vi "Pixy Logic Core.vi"() -> ()   [LabVIEW 2016]
uses:
  Robot Global Data.vi
panel:
  out "Lcal Pixy Out (Y Axis)":dbl(graph)=25.833333333333332
  out "Value Rejection History":i16(graph)=1
  in  "Past array Width":dbl[](array[numeric])=[26.0, 26.0, 26.0, 25.0, 26.0, 26.0]
  in  "Y Axis Range":dbl=100.0
  out "Lcal Pixy Out (X Axis)":dbl(graph)=25.833333333333332
  # "Decoded Pixy Outputs are located in\n    \"Pixy1Or2ObjectSelection.vi\""
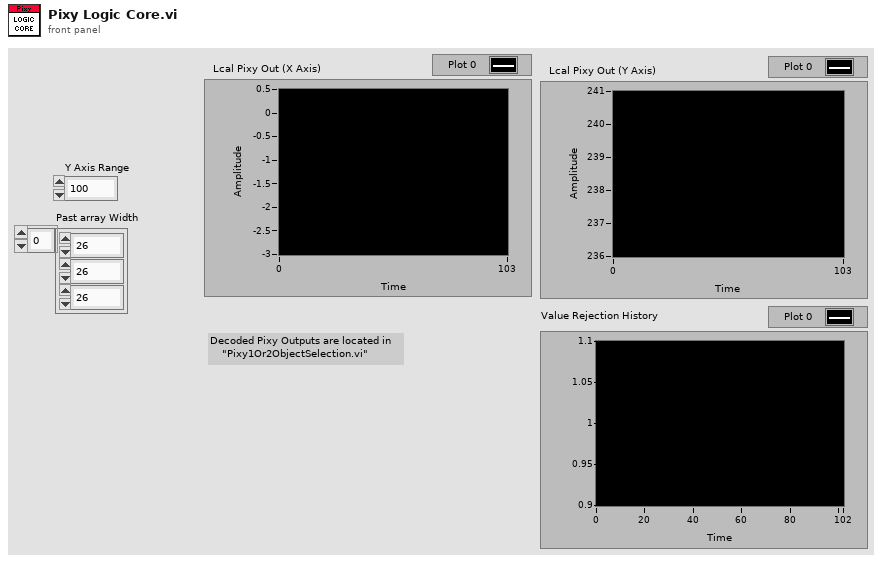
[diagram p1: front panel]
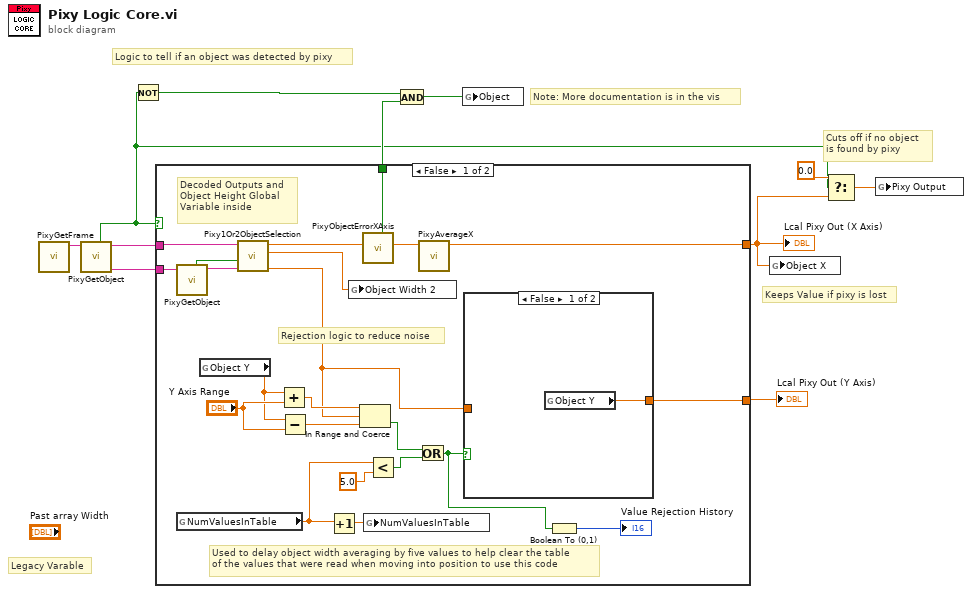
[diagram p0: block diagram]
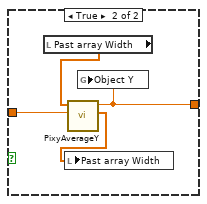
[diagram p2: hidden frame]
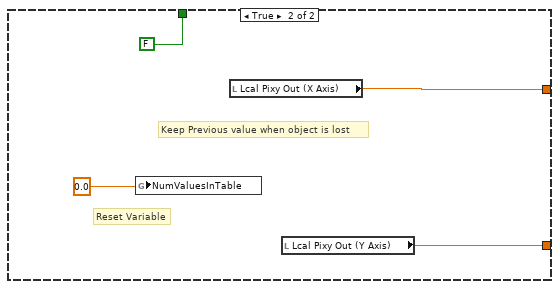
[diagram p3: hidden frame]
diagram:
  # "Note: More documentation is in the vis"
  # "Logic to tell if an object was detected by pixy"
  # "Legacy Varable"
  # "Keeps Value if pixy is lost"
  # "Cuts off if no object\nis found by pixy"
  n1 = call "PixyGetFrame.vi"() -> ("Frame"=w11:string)  [unwired: 11 in]
  n2 = call "PixyGetObject.vi"("Input Frame"=w11) -> ("Remainder of Frame"=w7:string, "Object"=w6:string, "Empty?"=w2:bool)  [unwired: 8 in]
  n3 = Not(x=w2) -> (.not. x?=w10:bool)
  n4 = case shown="False" w2 {
    tunnel: [w28 FALSE] -> w8
    tunnel: [w26 w41] -> w3
    tunnel: w7 -> [w33 _]
    tunnel: w6 -> [w30 _]
    tunnel: [w13 w39] -> w1
    frame False {
      # "Rejection logic to reduce noise"
      # "Used to delay object width averaging by five values to help clear the table\nof the values that were read when moving into position to use this code"
      # "Decoded Outputs and\nObject Height Global\nVariable inside"
      n5 = call "PixyGetObject.vi"("Input Frame"=w33) -> ("Object"=w31:string, "Empty?"=w32:bool)  [unwired: 8 in, 1 out]
      n6 = global read "Robot Global Data.vi" "NumValuesInTable"() -> (w22:dbl)
      n7 = global read "Robot Global Data.vi" "Object Y"() -> (w17:dbl)
      n8 = call "Pixy1Or2ObjectSelection.vi"("Second Object"=w31, "Empty?"=w32, "First Object"=w30) -> ("Y Axis Out"=w16:dbl, "Width Out"=w12:dbl, "X Axis Out"=w29:dbl)  [unwired: 6 in]
      n9 = Add(x=w17, y="Y Axis Range") -> (x+y=w20:dbl)
      n10 = Subtract(x=w17, y="Y Axis Range") -> (x-y=w19:dbl)
      n11 = Increment(x=w22) -> (x+1=w23:dbl)
      n12 = global write "Robot Global Data.vi" "Object Width 2"(w12) -> ()
      n13 = In Range and Coerce(upper limit=w20, x=w16, lower limit=w19) -> (In Range?=w21:bool)  [unwired: 1 out]
      n14 = call "PixyObjectErrorXAxis.vi"("Input Value"=w29) -> ("Output"=w27:dbl, "Object In Parameters"=w28:bool)  [unwired: 9 in]
      n15 = global write "Robot Global Data.vi" "NumValuesInTable"(w23) -> ()
      n16 = Less?(x=w22, y=5.0) -> (x < y?=w25:bool)
      n17 = Or(x=w21, y=w25) -> (x .or. y?=w14:bool)
      n18 = call "PixyAverageX.vi"("Input"=w27) -> ("mean"=w26:dbl)  [unwired: 10 in]
      n19 = case shown="False" w14 {
        tunnel: w16 -> [_ w36]
        tunnel: [w34 w35] -> w13
        frame False {
          n20 = global read "Robot Global Data.vi" "Object Y"() -> (w34:dbl)
        }
        frame True {
          n21 = local read "Past array Width"() -> (w37:dbl[])
          n22 = call "PixyAverageY.vi"("Input"=w36, "Past array Width"=w37) -> ("Array"=w38:dbl[], "mean"=w35:dbl)  [unwired: 8 in]
          n23 = local write "Past array Width"(w38) -> ()
          n24 = global write "Robot Global Data.vi" "Object Y"(w35) -> ()
        }
      }
      n25 = Boolean To (0,1)(Boolean=w14) -> (0, 1=→"Value Rejection History":i16)
    }
    frame True {
      # "Reset Variable"
      # "Keep Previous value when object is lost"
      n26 = global write "Robot Global Data.vi" "NumValuesInTable"(0.0 ("Height")) -> ()
      n27 = local read "Lcal Pixy Out (X Axis)"() -> (w41:dbl)
      n28 = local read "Lcal Pixy Out (Y Axis)"() -> (w39:dbl)
    }
  }
  "Lcal Pixy Out (X Axis)" <- w3
  "Lcal Pixy Out (Y Axis)" <- w1
  n29 = And(x=w10, y=w8) -> (x .and. y?=w9:bool)
  n30 = global write "Robot Global Data.vi" "Object"(w9) -> ()
  n31 = global write "Robot Global Data.vi" "Object X"(w3) -> ()
  n32 = Select(t=0.0, s=w2, f=w3) -> (s? t:f=w4:dbl)
  n33 = global write "Robot Global Data.vi" "Pixy Output"(w4) -> ()
